vi "boont_trig_test.vi"() -> ()   [LabVIEW 2015]
panel:
  in  "Signal Threshold":dbl
  in  "Signal Amplitude":dbl
  out "Signal State":bool
  in  "STOP":bool
  out "error out":errorcluster
  in  "error in (no error)":errorcluster
  in  "VISA Boonton":refnum<visa-resource-name>
  in  "VISA Scope":refnum<visa-resource-name>
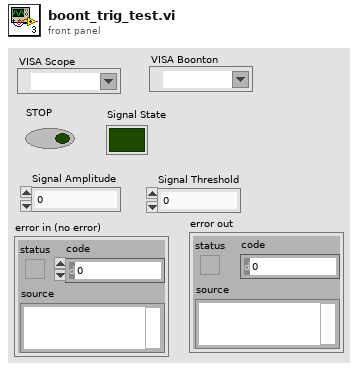
[diagram p1: front panel]
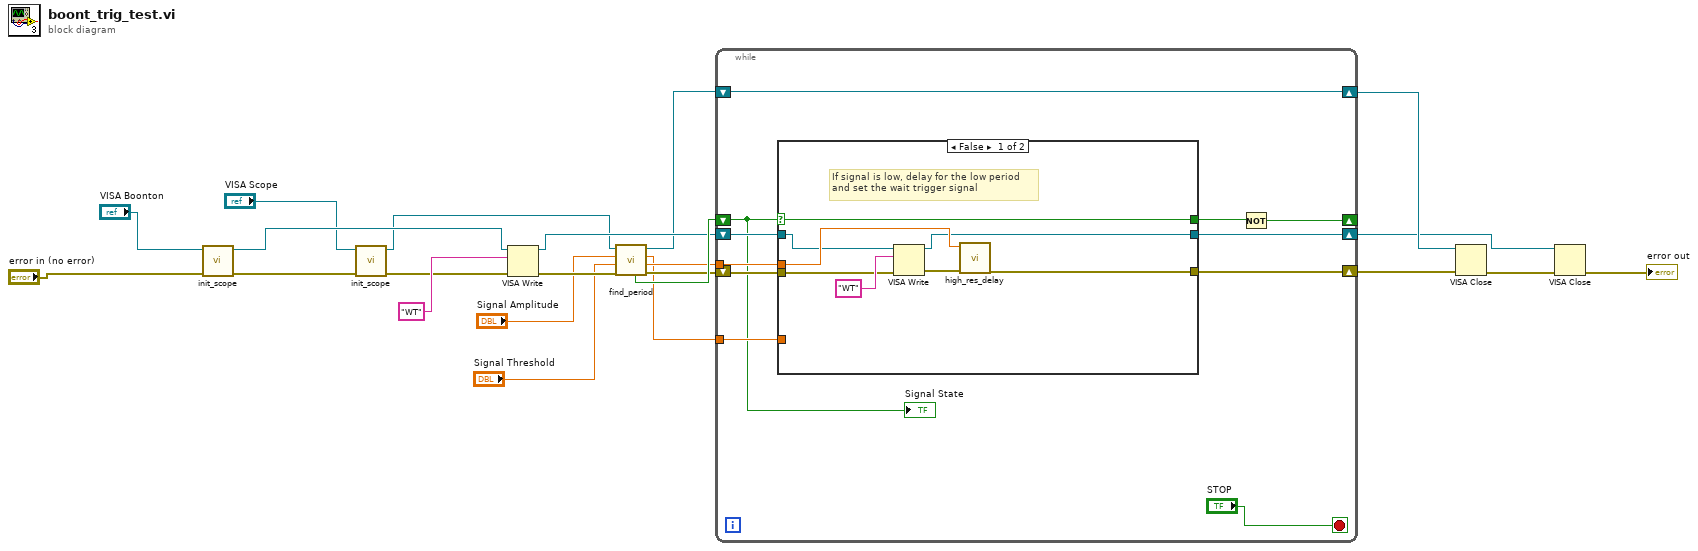
[diagram p0: block diagram]
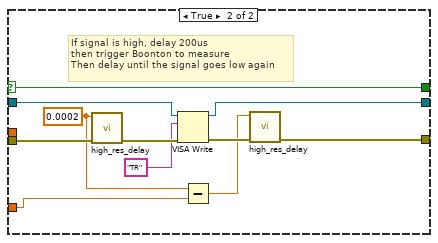
[diagram p2: hidden frame]
diagram:
  n1 = call "init_scope.vi"("error in (no error)"="error in (no error)", "VISA Scope"="VISA Boonton") -> ("error out"=w14:errorcluster, "VISA Scope Out"=w13:refnum<visa-resource-name>)  [unwired: 8 in]
  n2 = call "init_scope.vi"("error in (no error)"=w14, "VISA Scope"="VISA Scope") -> ("error out"=w15:errorcluster, "VISA Scope Out"=w12:refnum<visa-resource-name>)  [unwired: 8 in]
  n3 = VISA Write(VISA resource name=w13, write buffer="WT", error in (no error)=w15) -> (VISA resource name out=w17:refnum<visa-resource-name>, error out=w19:errorcluster)  [unwired: 1 out]
  n4 = call "find_period.vi"("error in (no error)"=w19, "Amplitude Thresh"="Signal Threshold", "Amplitude"="Signal Amplitude", "VISA In"=w12) -> ("error out"=w20:errorcluster, "Time Low"=w21:dbl, "Time High"=w16:dbl, "VISA Out"=w9:refnum<visa-resource-name>, "Pulse Status"=w22:bool)  [unwired: 2 in, 1 out]
  n5 = while {
    tunnel: w21 -> [w33]
    shift-right: [w29] -> _
    shift-left: w22 -> [w24]
    tunnel: w16 -> [w28]
    shift-right: [w27] -> w5
    shift-left: w17 -> [w31]
    shift-right: [w26] -> w7
    shift-left: w20 -> [w32]
    shift-right: [w25] -> w8
    shift-left: w9 -> [w25]
    stop <- "STOP" stop-if-true
    n6 = case shown="False" w24 {
      selector: w24 -> [w40 w51]
      tunnel: w33 -> [w37 _]
      tunnel: w32 -> [w39 w52]
      tunnel: [w40 w51] -> w30
      tunnel: w31 -> [w36 w49]
      tunnel: w28 -> [_ w46]
      tunnel: [w35 w43] -> w27
      tunnel: [w34 w42] -> w26
      frame False {
        # "If signal is low, delay for the low period\nand set the wait trigger signal"
        n7 = VISA Write(VISA resource name=w36, write buffer="WT", error in (no error)=w39) -> (VISA resource name out=w35:refnum<visa-resource-name>, error out=w38:errorcluster)  [unwired: 1 out]
        n8 = call "high_res_delay.vi"("error in (no error)"=w38, "Delay (sec)"=w37) -> ("error out"=w34:errorcluster)  [unwired: 9 in]
      }
      frame True {
        w47 = 0.0002 ("Delay (sec)")
        # "If signal is high, delay 200us\nthen trigger Boonton to measure\nThen delay until the signal goes low again"
        n9 = call "high_res_delay.vi"("error in (no error)"=w52, "Delay (sec)"=w47) -> ("error out"=w50:errorcluster)  [unwired: 9 in]
        n10 = VISA Write(VISA resource name=w49, write buffer="TR", error in (no error)=w50) -> (VISA resource name out=w43:refnum<visa-resource-name>, error out=w45:errorcluster)  [unwired: 1 out]
        n11 = Subtract(x=w47, y=w46) -> (x-y=w44:dbl)
        n12 = call "high_res_delay.vi"("error in (no error)"=w45, "Delay (sec)"=w44) -> ("error out"=w42:errorcluster)  [unwired: 9 in]
      }
    }
    n13 = Not(x=w30) -> (.not. x?=w29:bool)
    "Signal State" <- w24
  }
  n14 = VISA Close(VISA resource name=w8, error in (no error)=w7) -> (error out=w6:errorcluster)
  n15 = VISA Close(VISA resource name=w5, error in (no error)=w6) -> (error out=→"error out":errorcluster)
